vi "kvCanOpenChannel.vi"(0 "CAN Channel Number":u32, 1 "WantExclusive":bool, 2 "Override Exclusive":bool, 3 "AcceptVirtual":bool, 5 "WantExtended":bool, 7 "Accept Large DLC":bool, 9 "CAN FD":bool, 11 "error in (no error)":errorcluster, 12 "CAN FD NONISO":bool, 13 "No Init Access":bool, 14 "Require Init Access":bool) -> (4 "Opened Channel Handle\n(output only)":i32, 15 "error out":errorcluster)   [LabVIEW 2022 SP3]
doc: "Opens a CAN channel (circuit) and returns a handle which is used in subsequent calls to CANLIB."
uses:
  canlib32.dll
panel:
  # "Open Channel Flags"
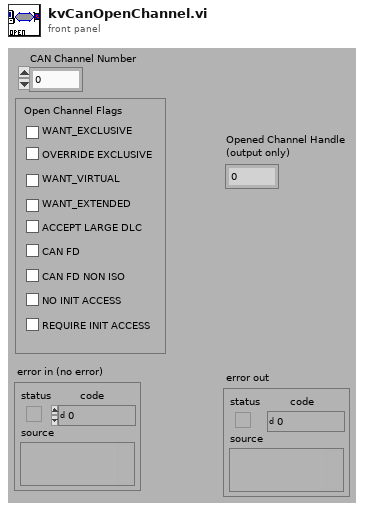
[diagram p1: front panel]
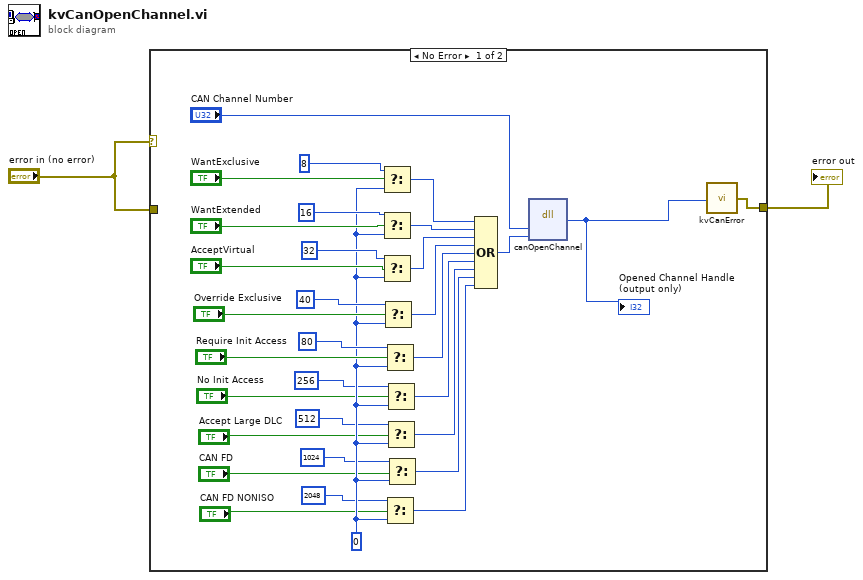
[diagram p0: block diagram]
diagram:
  n1 = case shown="No Error" "error in (no error)" {
    tunnel: [w24 w35] -> w2
    tunnel: "error in (no error)" -> [_ w35]
    frame No Error {
      w15 = u32 0
      n2 = Select(t=u32 8, s="WantExclusive", f=w15) -> (s? t:f=w28:u32)
      n3 = Select(t=u32 16, s="WantExtended", f=w15) -> (s? t:f=w27:u32)
      n4 = Select(t=u32 32, s="AcceptVirtual", f=w15) -> (s? t:f=w26:u32)
      n5 = Select(t=u32 40, s="Override Exclusive", f=w15) -> (s? t:f=w21:u32)
      n6 = Select(t=u32 80, s="Require Init Access", f=w15) -> (s? t:f=w20:u32)
      n7 = Select(t=u32 2048, s="CAN FD NONISO", f=w15) -> (s? t:f=w11:u32)
      n8 = Select(t=u32 256, s="No Init Access", f=w15) -> (s? t:f=w14:u32)
      n9 = Select(t=u32 512, s="Accept Large DLC", f=w15) -> (s? t:f=w13:u32)
      n10 = Select(t=u32 1024, s="CAN FD", f=w15) -> (s? t:f=w12:u32)
      n11 = Compound Arithmetic op=OR(w28, w27, w26, w21, w20, w14, w13, w12, w11) -> (w22:u32)
      n12 = dll-call lib="canlib32.dll" fn="canOpenChannel" label="Call Library Function"("channelNumber"="CAN Channel Number", "flags"=w22) -> (w23:i32)  [unwired: 5 in, 2 out]
      "Opened Channel Handle\n(output only)" <- w23
      n13 = call "kvCanError.vi"("error code"=w23) -> ("error out"=w24:errorcluster)
    }
    frame Error {
    }
  }
  "error out" <- w2
